vi "LVClass_WavefrontCorrector Get Current Preferences.vi"(0 "WavefrontCorrector in":refnum<class "WavefrontCorrector.lvclass">, 11 "error in (no error)":errorcluster) -> (4 "WavefrontCorrector out":refnum<class "WavefrontCorrector.lvclass">, 6 "sleep_after_movement":i32, 8 "Mirror preferences.Wavefront Corrector State":T1[](array[typedef]), 15 "error out":errorcluster)   [LabVIEW 2020, in "WavefrontCorrector.lvclass"]
doc: "Get current preferences.\n\n--------------------------------------------------------------------------------\n\n<B>correctorIn </B> : WavefrontCorrector object.\n<B>correctorOut </B> : WavefrontCorrector object.\n<B>sleep_after_movement </B> : WavefrontCorrector preferences : Time to stabilization (ms).\n<B>min </B> : WavefrontCorrector preferences : lowest command value.\n<B>max </B> : WavefrontCorrector preferences : highest command value.\n<B>validity </B> : WavefrontCorrector preferences : status.\n<B>fixed_values </B> : WavefrontCorrector preferences : fixed positions.\n<B>ErrorIn </B> : Error\n<B>ErrorOut </B> : Error\n\n--------------------------------------------------------------------------------"
uses:
  WavefrontCorrector.lvclass
  Wavefront Corrector states - ONE.ctl
  WavefrontCorrector.lvclass/WavefrontCorrector.ctl
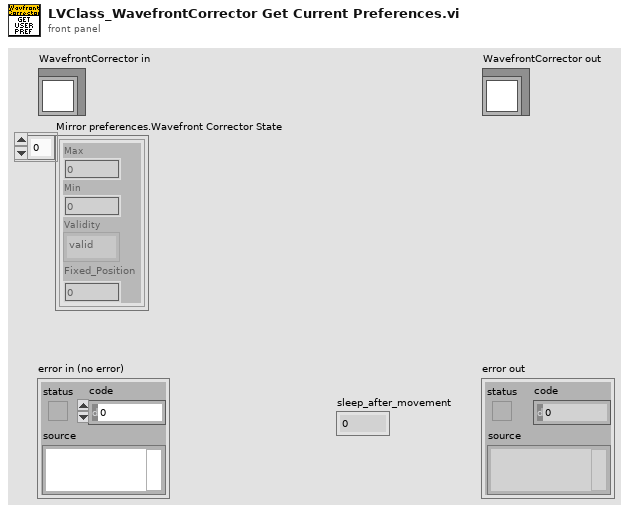
[diagram p1: front panel]
types:
  T1 = typedef "Wavefront Corrector states - ONE.ctl" = cluster{"Max":sgl, "Min":sgl, "Validity":enum16{"valid", "fixed", "invalid"}, "Fixed_Position":sgl}
  T2 = typedef "ClassID.ctl" = i64
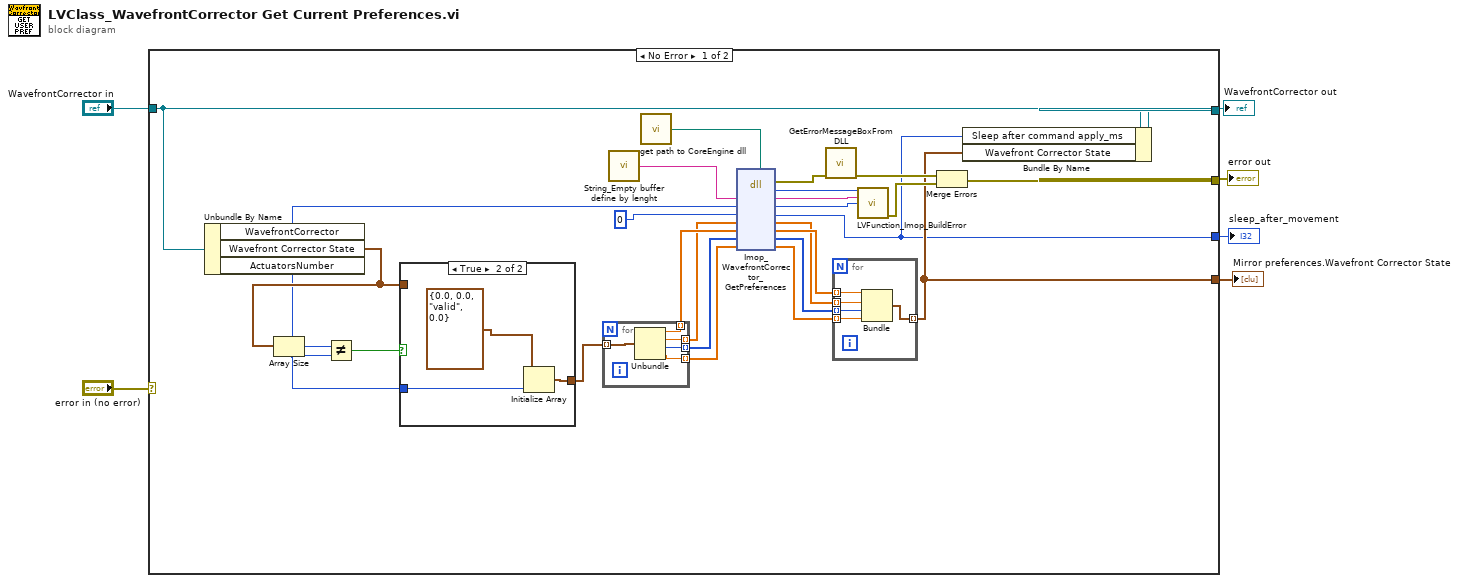
[diagram p0: block diagram]
diagram:
  n1 = case shown="No Error" "error in (no error)" {
    selector: "error in (no error)" -> [_ w50]
    tunnel: [w27 w50] -> w3
    tunnel: [w12 w49] -> w4
    tunnel: "WavefrontCorrector in" -> [w13 w49]
    tunnel: [w8 _] -> w2
    tunnel: [w9 _] -> w1
    frame No Error {
      n2 = Unbundle By Name(w13) -> ("WavefrontCorrector"=w21:T2, "Wavefront Corrector State"=w17:T1[], "ActuatorsNumber"=w11:i32)
      n3 = Array Size(array=w17) -> (size(s)=w19:i32)
      n4 = Not Equal?(x=w19, y=w11) -> (x != y?=w20:bool)
      n5 = case shown="True" w20 {
        tunnel: [w40 w43] -> w10
        tunnel: w11 -> [_ w42]
        tunnel: w17 -> [w40 _]
        frame False {
        }
        frame True {
          n6 = Initialize Array(T1 {"Max"=0.0, "Min"=0.0, "Validity"=enum."valid", "Fixed_Position"=0.0} ("Actuator state"), w42) -> (w43:T1[])
        }
      }
      n7 = for {
        tunnel: [w39] -> w18 mode=indexing
        tunnel: [w38] -> w16 mode=indexing
        tunnel: [w37] -> w15 mode=indexing
        tunnel: [w36] -> w14 mode=indexing
        tunnel: w10 -> [w35] mode=indexing
        n8 = Unbundle(w35) -> ("Max"=w39:sgl, "Min"=w38:sgl, "Validity"=w37:enum16{"valid", "fixed", "invalid"}, "Fixed_Position"=w36:sgl)
      }
      n9 = call "String_Empty buffer define by lenght.vi"() -> ("Empty buffer"=w32:string)  [unwired: 1 in]
      n10 = call "get path to CoreEngine dll.vi"() -> ("path to wavekit library"=w31:path)  [unwired: 14 in, 1 out]
      n11 = dll-call lib="D:/soft/HASO_v3/SVN_trunk/ImOpCoreEngine4_LV2011/DLLs/c_interface_vc100.dll" fn="Imop_WavefrontCorrector_GetPreferences"(path in=w31, "message"=w32, "WavefrontCorrection"=w21, "sleep_after_movement"=0, "min"=w16, "max"=w18, "validity"=w15, "fixed_value"=w14) -> (error out=w30:errorcluster, "return type"=w34:i32, "message"=w33:string, "WavefrontCorrection"=w7:i64, "sleep_after_movement"=w8:i32, "min"=w25:sgl[], "max"=w26:sgl[], "validity"=w24:i32[], "fixed_value"=w23:sgl[])  [unwired: 2 in, 1 out]
      n12 = call "GetErrorMessageBoxFromDLL.vi"("error IN"=w30) -> ("error OUT"=w29:errorcluster)  [unwired: 10 in]
      n13 = for {
        tunnel: w26 -> [w48] mode=indexing
        tunnel: w25 -> [w47] mode=indexing
        tunnel: w24 -> [w46] mode=indexing
        tunnel: w23 -> [w45] mode=indexing
        tunnel: [w44] -> w9 mode=indexing
        n14 = Bundle(w48, w47, w46, w45) -> (w44:cluster{sgl, sgl, i32, sgl})  [unwired: 1 in]
      }
      n15 = call "LVFunction_Imop_BuildError.vi"("code"=w34, "String to Prepend to source (\"\")"=w33, "Adresse"=w7) -> ("error out"=w28:errorcluster)  [unwired: 12 in]
      n16 = Merge Errors(w29, w28) -> (w27:errorcluster)
      n17 = Bundle By Name(cluster=w13, "Sleep after command apply_ms"=w8, "Wavefront Corrector State"=w9) -> (w12:refnum<class "WavefrontCorrector.lvclass">)
    }
    frame Error {
    }
  }
  "error out" <- w3
  "WavefrontCorrector out" <- w4
  "sleep_after_movement" <- w2
  "Mirror preferences.Wavefront Corrector State" <- w1
